vi "SCCAPI Is File In Local Path.vi"(8 "error in (no error)":errorcluster, 10 "files":path[](array[path]), 11 "source control reference in":T1) -> (0 "error out":errorcluster, 2 "in local path?":bool[](array[boolean]), 3 "source control reference out":T1)   [LabVIEW 2017, in "NI_SCC.lvlib"]
uses:
  <vilib>/SourceControl/sccapi/NI_SCC.lvlib
  <vilib>/SourceControl/sccapi/SCCAPI Refnum.ctl
  <vilib>/SourceControl/sccapi/SCCAPI SCC Operations.ctl
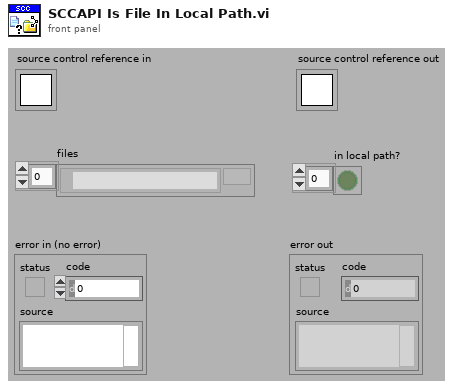
[diagram p1: front panel]
types:
  T1 = typedef "NI_SCC.lvlib/SCCAPI Refnum.ctl" = refnum<k1>
  T2 = typedef "NI_SCC.lvlib/SCCAPI SCC Operations.ctl" = enum16{"Add", "Check In", "Check Out", "Close Project", "Compare Files", "Compare VIs", "Configure Project", "File History", "File Properties", "File Status", "Find All Providers", "Get Advanced Command Options", "Get File Copy", "Get Latest Version", "Get Project Name", "Get StaticVI Path", "Initialize", "Not A Source Control Reference", "Open Project", "Provider Supports Functionality", "Remove", "Run Provider", "Undo Check Out", "Uninitialize", "Is File In Local Path"}
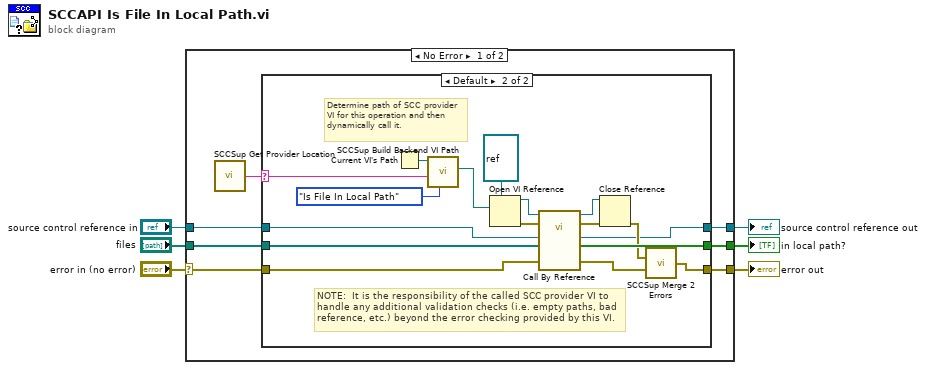
[diagram p0: block diagram]
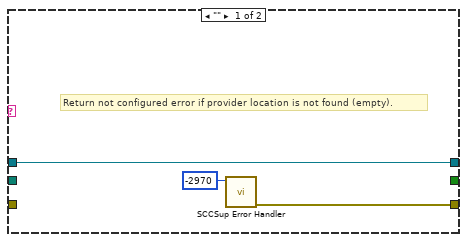
[diagram p2: hidden frame]
diagram:
  n1 = case shown="No Error" "error in (no error)" {
    selector: "error in (no error)" -> [w9 w35]
    tunnel: [w13 w35] -> w5
    tunnel: [w12 _] -> w3
    tunnel: "files" -> [w11 _]
    tunnel: "source control reference in" -> [w8 w34]
    tunnel: [w7 w34] -> w1
    frame No Error {
      n2 = call <vilib>:"SCCSup Get Provider Location.vi"() -> ("provider location"=w10:string)  [unwired: 6 in]
      n3 = case shown="Default" w10 {
        selector: w10 -> [_ w20]
        tunnel: [w15 w33] -> w13
        tunnel: [_ w27] -> w12
        tunnel: w11 -> [_ w26]
        tunnel: w9 -> [_ w19]
        tunnel: w8 -> [w14 w18]
        tunnel: [w14 w17] -> w7
        frame "" {
          # "Return not configured error if provider location is not found (empty)."
          n4 = call <vilib>:"SCCSup Error Handler.vi"("scc error code"=-2970 ("code")) -> ("error out"=w15:errorcluster)  [unwired: 10 in]
        }
        frame Default {
          # "NOTE:  It is the responsibility of the called SCC provider VI to handle any additional validation checks (i.e. empty paths, bad reference, etc.) beyond the error checking provided by this VI."
          # "Determine path of SCC provider VI for this operation and then dynamically call it."
          n5 = Current VI's Path() -> (path=w21:path)
          n6 = call <vilib>:"SCCSup Build Backend VI Path.vi"("scc operation"=SCCAPI_SCC_Operations."Is File In Local Path", "provider location"=w20, "caller path"=w21) -> ("scc backend VI path"=w23:path)  [unwired: 8 in]
          n7 = Open VI Reference(type specifier VI Refnum (for type only)=refnum<vi> refnum, vi path=w23) -> (vi reference=w31:refnum<vi>, error out=w30:errorcluster)  [unwired: 4 in]
          n8 = call-by-ref "?"(reference=w31, error in=w30, "error in (no error)"=w19, "files"=w26, "source control reference in"=w18) -> (reference out=w29:refnum<vi>, error out=w28:errorcluster, 0:"error out"=w24:errorcluster, "in local path?"=w27:bool[], "source control reference out"=w17:T1)  [unwired: 6 in]
          n9 = Close Reference(reference=w29, error in (no error)=w28) -> (error out=w25:errorcluster)
          n10 = call <vilib>:"SCCSup Merge 2 Errors.vi"("Error IO 1"=w25, "Error IO 2"=w24) -> ("Error IO out"=w33:errorcluster)  [unwired: 13 in]
        }
      }
    }
    frame Error {
    }
  }
  "error out" <- w5
  "in local path?" <- w3
  "source control reference out" <- w1
